vi "Complex Halfband Interpolator - 8spc.vi"(0 "input data":T1(array[cluster])=[{"I"=0.0, "Q"=0.0, "overflow"=FALSE}, {"I"=0.0, "Q"=0.0, "overflow"=FALSE}, {"I"=0.0, "Q"=0.0, "overflow"=FALSE}, {"I"=0.0, "Q"=0.0, "overflow"=FALSE}, {"I"=0.0, "Q"=0.0, "overflow"=FALSE}, {"I"=0.0, "Q"=0.0, "overflow"=FALSE}, {"I"=0.0, "Q"=0.0, "overflow"=FALSE}, {"I"=0.0, "Q"=0.0, "overflow"=FALSE}]) -> (4 "output data":T1(array[cluster]))   [LabVIEW 2019]
types:
  T1 = cluster{"I":fxp<+/-,18,1>, "Q":fxp<+/-,18,1>, "overflow":bool}[]
  T2 = cluster{"I":fxp<+/-,18,1>, "Q":fxp<+/-,18,1>, "overflow":bool}
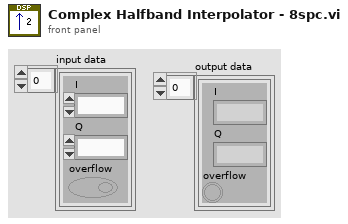
[diagram p1: front panel]
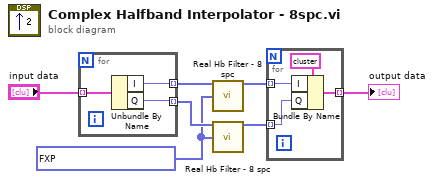
[diagram p0: block diagram]
diagram:
  w4 = fxp<+/-,18,1>[] [-0.00127410888671875, 0.00325775146484375, -0.0070953369140625, 0.01354217529296875, -0.02376556396484375, 0.03955841064453125, -0.0644073486328125, 0.10701751708984375, -0.1994476318359375, 0.6322708129882812] ("coefficients")
  n1 = for {
    tunnel: "input data" -> [w10] mode=indexing
    tunnel: [w9] -> w6 mode=indexing
    tunnel: [w8] -> w5 mode=indexing
    n2 = Unbundle By Name(w10) -> ("I"=w9:fxp<+/-,18,1>, "Q"=w8:fxp<+/-,18,1>)
  }
  n3 = call "Real Hb Filter - 8 spc.vi"("input data"=w6, "coefficients"=w4) -> ("output data"=w3:fxp<+/-,18,1>[])  [unwired: 13 in]
  n4 = call "Real Hb Filter - 8 spc.vi"("input data"=w5, "coefficients"=w4) -> ("output data"=w2:fxp<+/-,18,1>[])  [unwired: 13 in]
  n5 = for {
    tunnel: w3 -> [w13] mode=indexing
    tunnel: w2 -> [w12] mode=indexing
    tunnel: [w11] -> w1 mode=indexing
    n6 = Bundle By Name(cluster=T2 {"I"=0.0, "Q"=0.0, "overflow"=FALSE} ("IQ Data"), "I"=w13, "Q"=w12) -> (w11:T2)
  }
  "output data" <- w1
